vi "Reset state.vi"(8 "error in (no error)":errorcluster, 11 "StateManager in":refnum<class "StateManager.lvclass">) -> (0 "error out":errorcluster, 3 "StateManager out":refnum<class "StateManager.lvclass">)   [LabVIEW 2018, in "StateManager.lvclass"]
uses:
  StateManager.lvclass
  StateManager.lvclass/StateManager.ctl
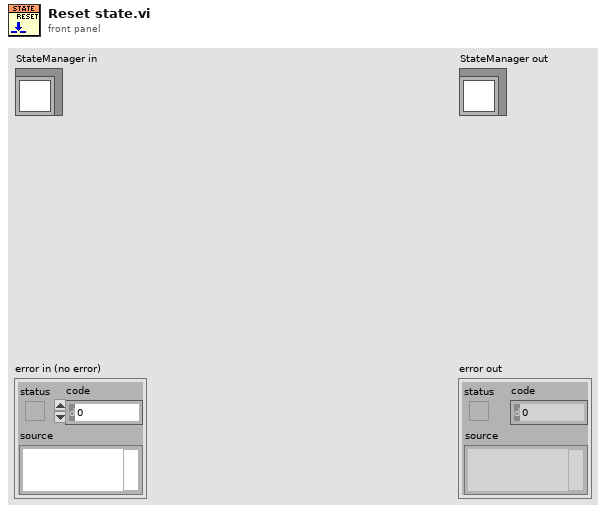
[diagram p1: front panel]
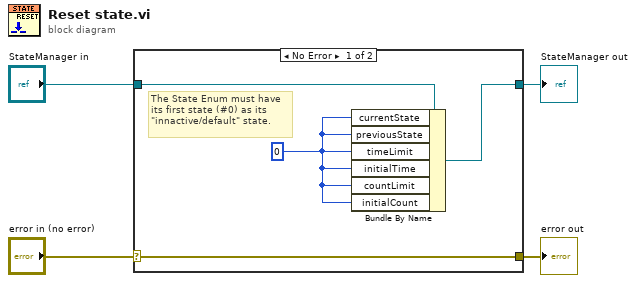
[diagram p0: block diagram]
diagram:
  n1 = case shown="No Error" "error in (no error)" {
    selector: "error in (no error)" -> [w8 w9]
    tunnel: [w8 w9] -> w3
    tunnel: [w6 w10] -> w1
    tunnel: "StateManager in" -> [w7 w10]
    frame No Error {
      w5 = u32 0 ("timeLimit")
      # "The State Enum must have\nits first state (#0) as its \n\"innactive/default\" state."
      n2 = Bundle By Name(cluster=w7, "currentState"=w5, "previousState"=w5, "timeLimit"=w5, "initialTime"=w5, "countLimit"=w5, "initialCount"=w5) -> (w6:refnum<class "StateManager.lvclass">)
    }
    frame Error {
    }
  }
  "error out" <- w3
  "StateManager out" <- w1
